vi "Parse_Command_Arguments.vi"(0 "Command String":string) -> (1 "Command":string, 2 "Argument List":string[](array[string]))   [LabVIEW 2011]
doc: "This VI parses a command string with its arguments. For example, an input string such as \"Command:Argument1,Argument2(\"some text\") would return a command value of \"Command\" and an argument list containing the discrete values \"Argument1\" and \"Argument2(\"some text\")\"."
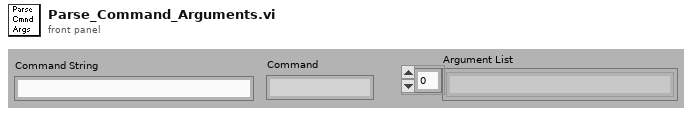
[diagram p1: front panel]
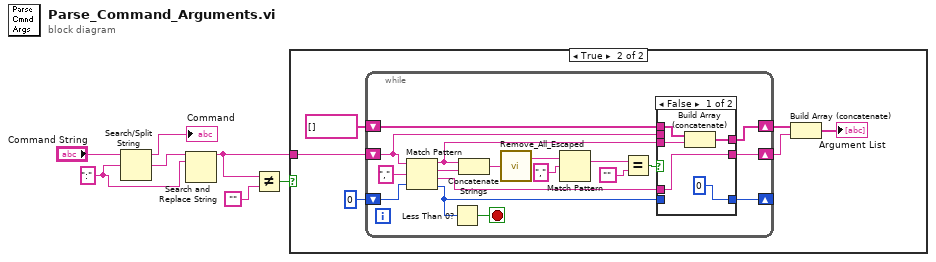
[diagram p0: block diagram]
diagram:
  w6 = ":" ("search string/char (-)")
  n1 = Search/Split String(string="Command String", search string/char (-)=w6) -> (substring before match=→"Command":string, match + rest of string=w4:string)  [unwired: 2 out]
  n2 = Search and Replace String(input string=w4, search string=w6) -> (result string=w1:string)  [unwired: 1 in, 8 out]
  n3 = Not Equal?(x=w1, y="") -> (x != y?=w3:bool)
  n4 = case shown="True" w3 {
    tunnel: w1 -> [_ w13]
    frame False {
    }
    frame True {
      n5 = while {
        shift-right: [w20] -> w9
        shift-left: w13 -> [w19]
        shift-right: [w22] -> w10
        shift-left: string[] [] -> [w24]
        shift-right: [w17] -> _
        shift-left: 0 ("offset past match") -> [w18]
        stop <- w15 stop-if-true
        n6 = Match Pattern(string=w19, regular expression=",", offset (0)=w18) -> (before substring=w23:string, match substring=w30:string, after substring=w14:string, offset past match=w16:i32)
        n7 = Less Than 0?(x=w16) -> (x < 0?=w15:bool)
        n8 = Concatenate Strings(w23, w30) -> (w29:string)
        n9 = call "Remove_All_Escaped.vi"("Input String"=w29) -> ("Output String"=w26:string)  [unwired: 1 out]
        n10 = Match Pattern(string=w26, regular expression=",") -> (match substring=w25:string)  [unwired: 1 in, 3 out]
        n11 = Equal?(x=w25, y="") -> (x = y?=w21:bool)
        n12 = case shown="False" w21 {
          tunnel: w24 -> [w36 w39]
          tunnel: w23 -> [w34 _]
          tunnel: [w35 w39] -> w22
          tunnel: [w32 w37] -> w20
          tunnel: w19 -> [_ w37]
          tunnel: w16 -> [_ w38]
          tunnel: [0 w38] -> w17
          tunnel: w14 -> [w32 _]
          frame False {
            n13 = Build Array (concatenate)(w36, w34) -> (w35:string[])
          }
          frame True {
          }
        }
      }
      n14 = Build Array (concatenate)(w10, w9) -> (→"Argument List":string[])
    }
  }
